vi "AlliGator Compute Weighted Phasor Plot Statistics.vi"(6 "Phasor Frequency":dbl[unit], 7 "Plot Name(s)":string, 8 "error in (no error)":errorcluster, 9 "Intensity Array":dbl[](array[numeric]), 10 "s Array":dbl[](array[numeric]), 11 "g Array":dbl[](array[numeric])) -> (0 "error out":errorcluster, 1 "Result String":string, 2 "Phasor SDV (g, s)":T1, 3 "Phasor (g, s)":T1)   [LabVIEW 2021, in "AlliGator Phasor Graph.lvlib"]
doc: "Computes the (intensity-weighted) average phasor, SDV and related quantities for a phasor array."
uses:
  AlliGator Phasor Graph.lvlib
  Phasor/Phasor (g, s).ctl
  Phasor/Phasor.lvlib
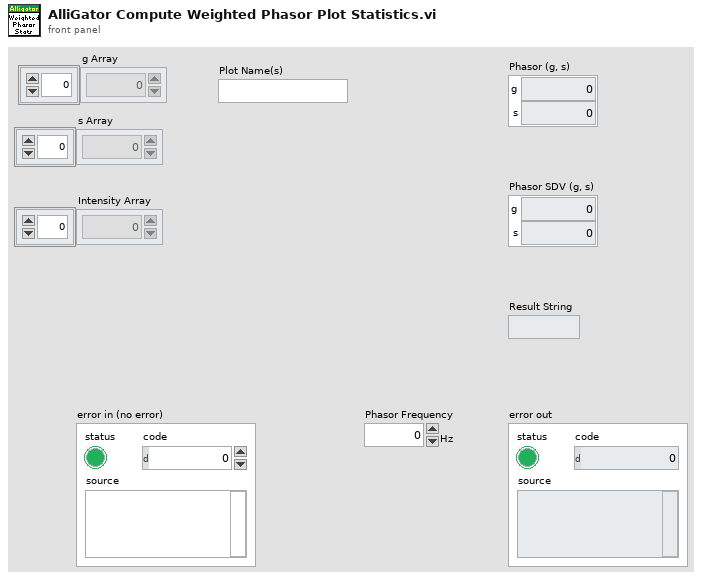
[diagram p1: front panel]
types:
  T1 = typedef "Phasor.lvlib/Phasor (g, s).ctl" = cluster{"g":dbl, "s":dbl}
  T2 = typedef "AlliGator Phasor Plot Statistics.ctl" = cluster{"Average g (weighted)":dbl, "g SDV (weighted)":dbl, "Average s (weighted)":dbl, "s SDV (weighted)":dbl, "Average tau_phi (weighted)":dbl, "tau_phi SDV (weighted)":dbl, "Average tau_m (weighted)":dbl, "tau_m SDV (weighted)":dbl, "Average Amplitude Ratio (weighted)":dbl, "Amplitude Ratio SDV (weighted)":dbl, "Amplitude-Averaged Lifetime (weighted)":dbl, "Amplitude-Averaged Lifetime SDV (weighted)":dbl, "Average Intensity Ratioweighted)":dbl, "Intensity Ratio SDV (weighted)":dbl, "Intensity-Averaged Lifetime (weighted)":dbl, "Intensity-Averaged Lifetime SDV (weighted)":dbl}
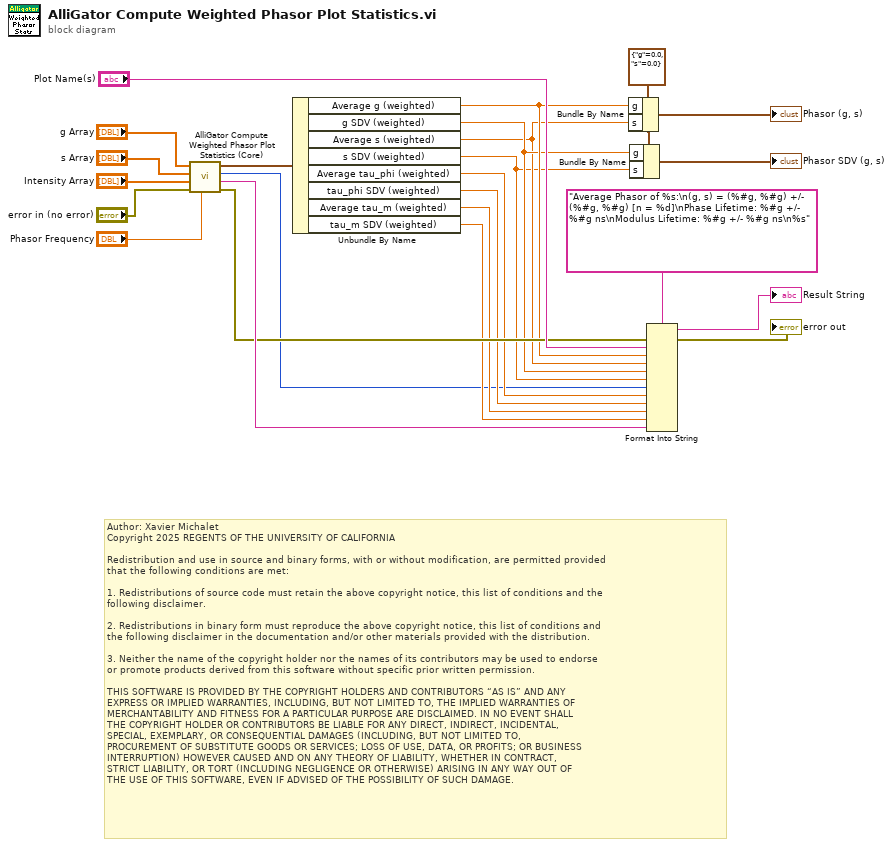
[diagram p0: block diagram]
diagram:
  w21 = T1 {"g"=0.0, "s"=0.0} ("Phasor (g, s)")
  # "Author: Xavier Michalet\nCopyright 2025 REGENTS OF THE UNIVERSITY OF CALIFORNIA\n\nRedistribution and use in source and binary forms, with or without modification, are permitted provided\nthat the following conditions are met:\n\n1. Redistributions of source code must retain the above copyright notice, this list of conditions and the\nfollowing disclaimer.\n\n2. Redistributions in binary form must reproduce the above copyright notice, this list of conditions and\nthe following disclaimer in the documentation and/or other materials provided with the distribution.\n\n3. Neither the name of the copyright holder nor the names of its contributors may be used to endorse \nor promote products derived from this software without specific prior written permission.\n\nTHIS SOFTWARE IS PROVIDED BY THE COPYRIGHT HOLDERS AND CONTRIBUTORS “AS IS” AND ANY \nEXPRESS OR IMPLIED WARRANTIES, INCLUDING, BUT NOT LIMITED TO, THE IMPLIED WARRANTIES OF\nMERCHANTABILITY AND FITNESS FOR A PARTICULAR PURPOSE ARE DISCLAIMED. IN NO EVENT SHALL\nTHE COPYRIGHT HOLDER OR CONTRIBUTORS BE LIABLE FOR ANY DIRECT, INDIRECT, INCIDENTAL, \nSPECIAL, EXEMPLARY, OR CONSEQUENTIAL DAMAGES (INCLUDING, BUT NOT LIMITED TO, \nPROCUREMENT OF SUBSTITUTE GOODS OR SERVICES; LOSS OF USE, DATA, OR PROFITS; OR BUSINESS\nINTERRUPTION) HOWEVER CAUSED AND ON ANY THEORY OF LIABILITY, WHETHER IN CONTRACT, \nSTRICT LIABILITY, OR TORT (INCLUDING NEGLIGENCE OR OTHERWISE) ARISING IN ANY WAY OUT OF\nTHE USE OF THIS SOFTWARE, EVEN IF ADVISED OF THE POSSIBILITY OF SUCH DAMAGE."
  n1 = call "AlliGator Compute Weighted Phasor Plot Statistics (Core).vi"("Phasor Frequency"="Phasor Frequency", "error in (no error)"="error in (no error)", "Intensity Array"="Intensity Array", "s Array"="s Array", "g Array"="g Array") -> ("error out"=w12:errorcluster, "String"=w13:string, "Effective # Elements"=w2:i32, "Phasor Plot Statistics"=w11:T2)  [unwired: 3 in]
  n2 = Unbundle By Name(w11) -> ("Average g (weighted)"=w10:dbl, "g SDV (weighted)"=w9:dbl, "Average s (weighted)"=w8:dbl, "s SDV (weighted)"=w7:dbl, "Average tau_phi (weighted)"=w6:dbl, "tau_phi SDV (weighted)"=w5:dbl, "Average tau_m (weighted)"=w4:dbl, "tau_m SDV (weighted)"=w3:dbl)
  n3 = Bundle By Name(cluster=w21, "g"=w10, "s"=w8) -> (→"Phasor (g, s)":T1)
  n4 = Bundle By Name(cluster=w21, "g"=w9, "s"=w7) -> (→"Phasor SDV (g, s)":T1)
  n5 = Format Into String(format string="Average Phasor of %s:\n(g, s) = (%#g, %#g) +/- (%#g, %#g) [n = %d]\nPhase Lifetime: %#g +/- %#g ns\nModulus Lifetime: %#g +/- %#g ns\n%s" ("initial string"), error in=w12, "Plot Name(s)", w10, w8, w9, w7, w2, w6, w5, w4, w3, w13) -> (resulting string=→"Result String":string, error out=→"error out":errorcluster)  [unwired: 1 in]
